vi "Avec de la chance.vi"() -> ()   [LabVIEW 2013]
panel:
  out "nombre d'iteration":dbl
  out "tirage actuel":dbl
  in  "Nombre à obtenir":u32 max=100000 step=1
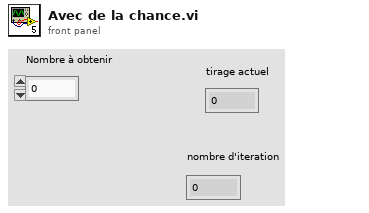
[diagram p1: front panel]
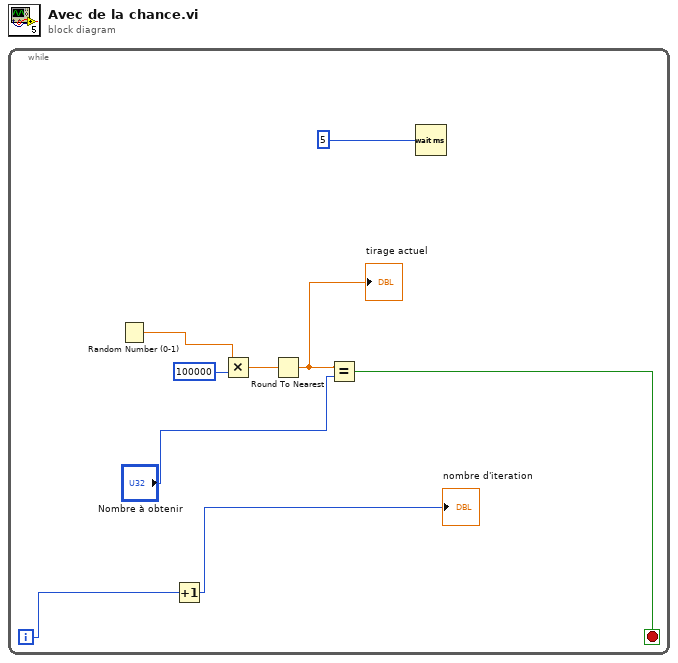
[diagram p0: block diagram]
diagram:
  n1 = while {
    i -> [w2]
    stop <- w6 stop-if-true
    n2 = Random Number (0-1)() -> (number: 0 to 1=w8:dbl)
    n3 = Increment(x=w2) -> (x+1=→"nombre d'iteration":i32)
    n4 = Multiply(x=w8, y=100000) -> (x*y=w5:dbl)
    n5 = Round To Nearest(number=w5) -> (nearest integer value=w4:dbl)
    "tirage actuel" <- w4
    n6 = Equal?(x=w4, y="Nombre à obtenir") -> (x = y?=w6:bool)
    n7 = Wait (ms)(milliseconds to wait=5) -> ()  [unwired: 1 out]
  }
